vi "QuickCast.vi"(8 "YActorIn":refnum<class>, 9 "ObjectTargetType":refnum<class>) -> (10 "ObjectOut":refnum<class>)   [LabVIEW 2021, in "YActor.lvclass"]
uses:
  YActor.lvclass
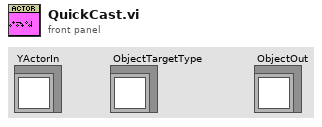
[diagram p1: front panel]
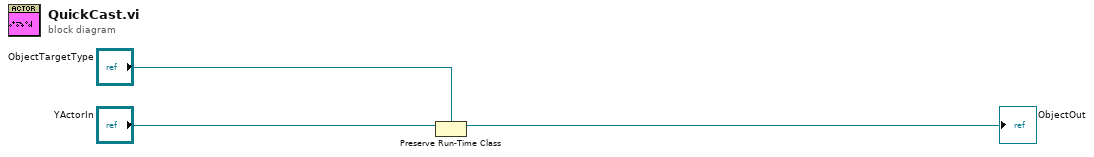
[diagram p0: block diagram]
diagram:
  n1 = Preserve Run-Time Class(object in="YActorIn", 2:"ObjectTargetType") -> (object out=→"ObjectOut":refnum<class>)  [unwired: 1 in, 1 out]
